vi "SaveXferFnData.vi"() -> ()   [LabVIEW 2016]
uses:
  Globals/Meas_global.vi
  Globals/Plug_in_data_global.vi
panel:
  in  "Name2":string="MyNameHere"
  in  "Name1":string="MyNameHere"
  in  "Inst name":string="MyNameHere"
  in  "XferFn":string[][](array[string])
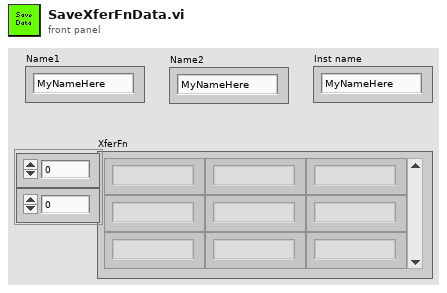
[diagram p1: front panel]
types:
  T1 = typedef "Post_Process.ctl" = enum16{"Take New Data", "Post Process Raw Data File"}
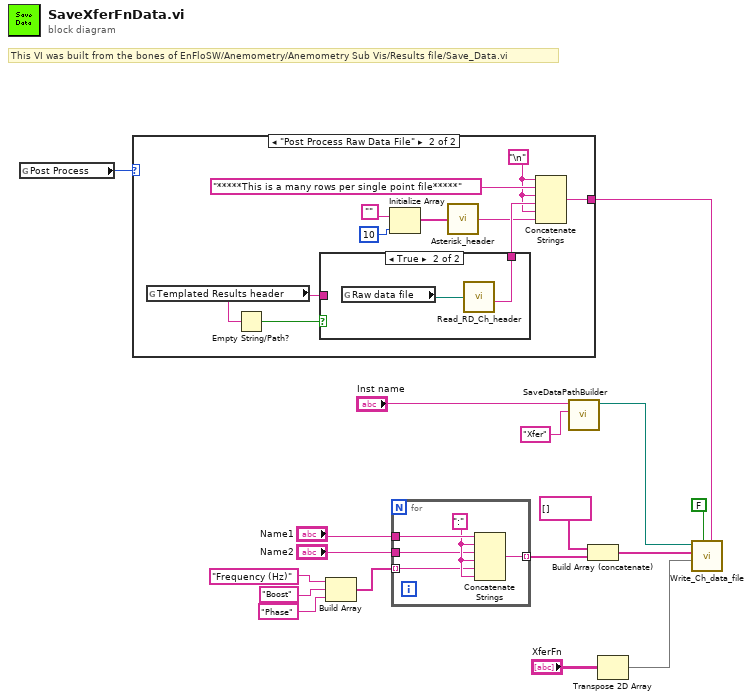
[diagram p0: block diagram]
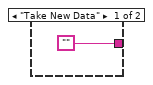
[diagram p2: hidden frame]
diagram:
  # "This VI was built from the bones of EnFloSW/Anemometry/Anemometry Sub Vis/Results file/Save_Data.vi"
  n1 = global read "Meas_global.vi" "Post Process"() -> (w17:T1)
  n2 = case shown="\"Post Process Raw Data File\"" w17 {
    tunnel: ["" w19] -> w5
    frame "Take New Data" {
    }
    frame "Post Process Raw Data File" {
      w20 = "\n"
      n3 = global read "Plug_in_data_global.vi" "Templated Results header"() -> (w25:string)
      n4 = Empty String/Path?(string/path=w25) -> (empty?=w27:bool)
      n5 = case shown="True" w27 {
        tunnel: [w29 w30] -> w26
        tunnel: w25 -> [w29 _]
        frame False {
        }
        frame True {
          n6 = global read "Meas_global.vi" "Raw data file"() -> (w31:path)
          n7 = call "Read_RD_Ch_header.vi"("Raw data file"=w31) -> ("Ch string"=w30:string)  [unwired: 3 out]
        }
      }
      n8 = Initialize Array("", 10) -> (w24:string[])
      n9 = call "Asterisk_header.vi"("Channel names"=w24) -> ("Header string"=w21:string)
      n10 = Concatenate Strings(w20, "*****This is a many rows per single point file*****", w20, w26, w20, w21) -> (w19:string)
    }
  }
  n11 = Build Array("Frequency (Hz)", "Boost", "Phase") -> (w11:string[])
  n12 = for {
    tunnel: "Name1" -> [w36]
    tunnel: "Name2" -> [w34]
    tunnel: [w33] -> w12 mode=indexing
    tunnel: w11 -> [w32] mode=indexing
    w35 = ":" ("string")
    n13 = Concatenate Strings(w36, w35, w34, w35, w32, w35) -> (w33:string)
  }
  n14 = call "SaveDataPathBuilder.vi"("DataTypeSuffix"="Xfer", "Inst name"="Inst name") -> ("Path name Out"=w13:path)  [unwired: 9 in]
  n15 = Build Array (concatenate)(string[] [], w12) -> (w15:string[])
  n16 = Transpose 2D Array(2D array="XferFn") -> (transposed array=w14:string[][])
  n17 = call "Write_Ch_data_file.vi"("Header string"=w5, "exists?"=FALSE, "Channel Values"=w14, "Channel names"=w15, "Filename"=w13) -> ()  [unwired: 2 in, 5 out]
